vi "Write Flattener.vi"(10 "Flattener":refnum<class "Message Flattener.lvclass">, 11 "TCP Stream in":refnum<class "TCP Stream.lvclass">) -> (3 "TCP Stream out":refnum<class "TCP Stream.lvclass">)   [LabVIEW 2020, in "TCP Stream.lvclass"]
doc: "Use this VI to set the message flattener to be used when reading or writing message."
uses:
  TCP Stream.lvclass
  Abstract Classes/Message Flattener/Message Flattener.lvclass
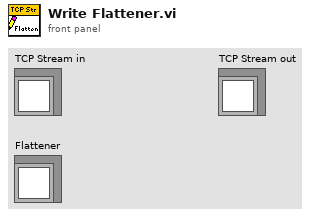
[diagram p1: front panel]
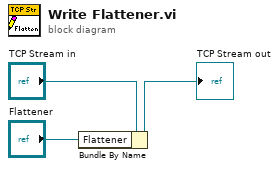
[diagram p0: block diagram]
diagram:
  n1 = Bundle By Name(cluster="TCP Stream in", "Flattener"="Flattener") -> (→"TCP Stream out":refnum<class "TCP Stream.lvclass">)
